vi "Get Auth URL.vi"(11 "OAuth2 in":refnum<class "OAuth2.lvclass">) -> (2 "Auth URL":string)   [LabVIEW 2020, in "OAuth2.lvlib" / "OAuth2.lvclass"]
uses:
  OAuth2.lvclass
  OAuth2.lvclass/OAuth2.ctl
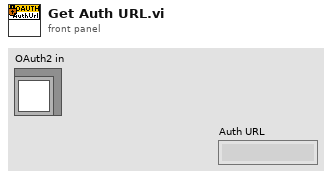
[diagram p1: front panel]
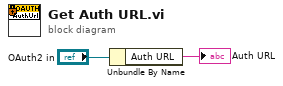
[diagram p0: block diagram]
diagram:
  n1 = Unbundle By Name("OAuth2 in") -> ("Auth URL"=→"Auth URL":string)
